vi "Query Sweep Time.vi"(7 "Sweep Time Param (sweep time)":T1, 8 "error in (no error)":errorcluster, 10 "Channel (0: Channel 1)":T2 items=["Channel 1", "Channel 2"], 11 "VISA resource name":refnum<visa-resource-name>) -> (0 "error out":errorcluster, 1 "time":dbl[unit], 3 "VISA resource name out":refnum<visa-resource-name>)   [LabVIEW 2009, in "Tektronix AFG 3000 Series.lvlib"]
doc: "Queries the sweep time, hold time (htime), or return time (rtime) of a Tektronix AFG 3000 series function generator. The sweep time does not include hold time and return time, and return time does not include hold time."
uses:
  Tektronix AFG 3000 Series.lvlib
  controls.llb/Channel.ctl
  controls.llb/Sweep Time Parameter.ctl
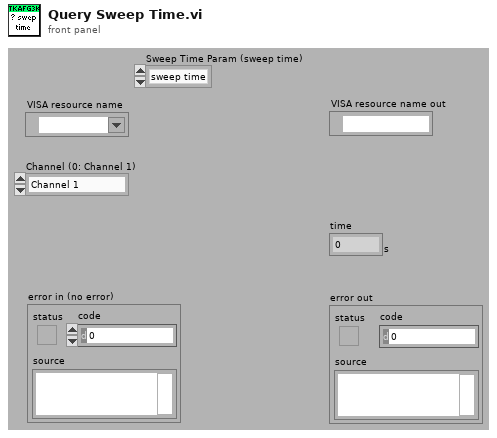
[diagram p1: front panel]
types:
  T1 = typedef "Sweep Time Parameter.ctl" = enum16{"sweep time", "hold time", "return time"}
  T2 = typedef "Channel.ctl" = u16
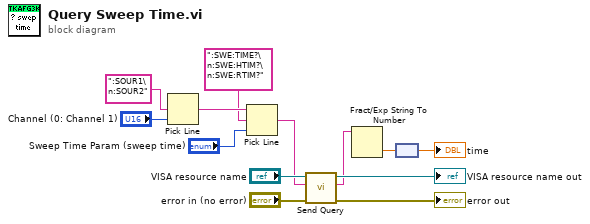
[diagram p0: block diagram]
diagram:
  n1 = Pick Line(multi-line string=":SOUR1\n:SOUR2", line index="Channel (0: Channel 1)") -> (output string=w4:string)  [unwired: 1 out]
  n2 = Pick Line(string ("")=w4, multi-line string=":SWE:TIME?\n:SWE:HTIM?\n:SWE:RTIM?", line index="Sweep Time Param (sweep time)") -> (output string=w1:string)
  n3 = call "Send Query.vi"("error in (no error)"="error in (no error)", "write buffer"=w1, "VISA resource name"="VISA resource name") -> ("error out"=→"error out":errorcluster, "read buffer"=w7:string, "VISA resource name out"=→"VISA resource name out":refnum<visa-resource-name>)  [unwired: 1 in, 5 out]
  n4 = Fract/Exp String To Number(string=w7) -> (number=w6:dbl)  [unwired: 4 out]
  n5 = node(w6) -> (→"time":dbl[unit])
